vi "LINX - Blink (Advanced).vi"() -> ()   [LabVIEW 2020]
doc: "Automatically blink and LED attached to a digital output channel of a LINX device."
uses:
  vi.lib/MakerHub/LINX/Public/Peripherals/Digital/Digital Write 1 Chan.vi
  vi.lib/MakerHub/LINX/Public/Peripherals/Digital/Digital Write N Chans.vi
  vi.lib/MakerHub/LINX/Private/Local IO/LinxDigitalWrite.vi
  vi.lib/MakerHub/LINX/Public/Utilities/Check Channel.vi
  vi.lib/MakerHub/LINX/Public/Utilities/Open Serial.vi
  vi.lib/MakerHub/LINX/Private/Utilties/Generate Error.vi
  vi.lib/MakerHub/LINX/LMH-LINX.lvlib
  vi.lib/MakerHub/LINX/Private/Device/Device.lvlib
panel:
  out "LED Value":bool
  in  "Digital Output Channel":u8=13
  in  "Serial Port":refnum<visa-resource-name>
  out "Loop Rate (Hz)":u32
  in  "Stop Button":bool
  # "Circuit Schematic"
  # "LINX Device Settings"
  # "LED Value"
  # "Blink (Serial Interface)\n\nThis example demonstrates how to blink an LED on a LINX device connected to \nthe host computer using USB / Serial.\n\nInstructions\n1. Select the Serial Port associated with the LINX Device.\n2. Select the Digital Pin connected to the LED.\n3. Click the Run Arrow."
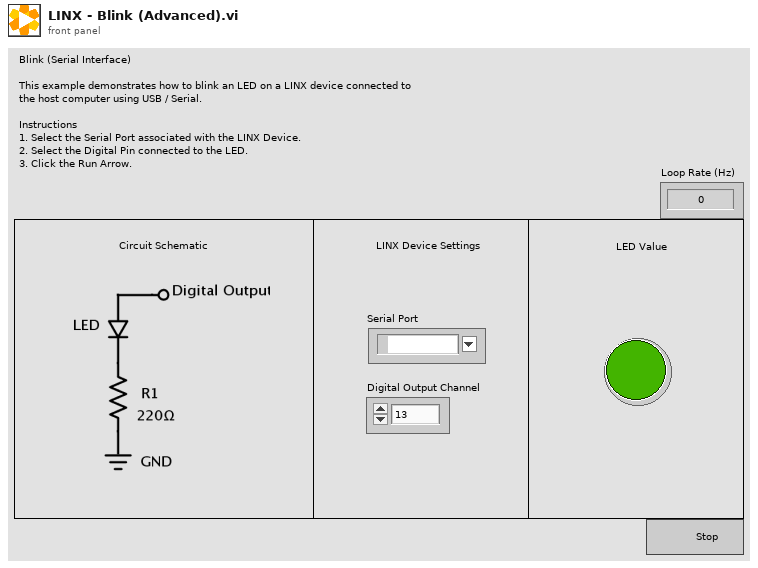
[diagram p1: front panel]
types:
  T1 = typedef "LMH-LINX.lvlib/LINX Ref.ctl" = cluster{"IO":T2, "Interface":T3, "LINX Device Config":T4}
  T2 = typedef "LMH-LINX.lvlib/Platform.ctl" = enum16{"Remote", "Local"}
  T3 = typedef "LMH-LINX.lvlib/Interface.ctl" = enum16{"Serial", "TCP"}
  T4 = typedef "Device.lvlib/LINX Device Config.ctl" = cluster{"Interface":T3, "COM Port":refnum<visa-resource-name>, "TCP Configuration":T5, "Device Family":u8, "Device ID":u8, "Device Name":string, "TCP Ref":refnum<k5>, "Channels":T6}
  T5 = typedef "Device.lvlib/TCP Config.ctl" = cluster{"IP Address":string, "Port":u16}
  T6 = typedef "LMH-LINX.lvlib/Channels.ctl" = cluster{"DI":u8[], "DO":u8[], "AI":u8[], "AO":u8[], "PWM":u8[], "QE":u8[], "UART":u8[], "I2C 2":u8[], "SPI":u8[], "CAN":u8[], "Servo":u8[], "AI Ref (V)":dbl, "AI Resolution (Bits)":u8, "AO Ref (V)":dbl, "AO Resolution (Bits)":u8}
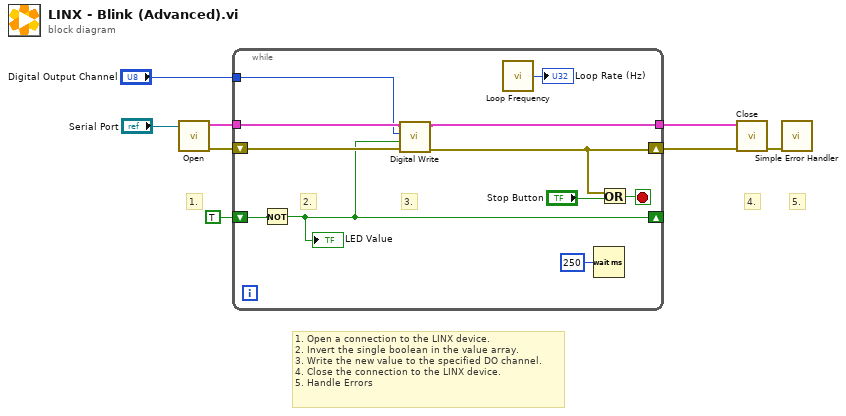
[diagram p0: block diagram]
diagram:
  # "1. Open a connection to the LINX device.\n2. Invert the single boolean in the value array.\n3. Write the new value to the specified DO channel.\n4. Close the connection to the LINX device.\n5. Handle Errors"
  # "5."
  # "4."
  # "1."
  n1 = call-poly "Open.vi"("Serial Port"="Serial Port") -> ("Error Out"=w7:errorcluster, "LINX Resource"=w8:T1)  [unwired: 8 in, 1 out]
  n2 = while {
    tunnel: w8 -> [w16]
    tunnel: [w15] -> w6
    shift-right: [w13] -> w5
    shift-left: w7 -> [w14]
    shift-right: [w9] -> _
    shift-left: TRUE -> [w10]
    tunnel: "Digital Output Channel" -> [w11]
    stop <- w19 stop-if-true
    # "2."
    # "3."
    n3 = Not(x=w10) -> (.not. x?=w9:bool)
    "LED Value" <- w9
    n4 = call-poly "Digital Write.vi"("Error In"=w14, "Output Value"=w9, "DO Channel"=w11, "LINX Resource"=w16) -> ("Error Out"=w13:errorcluster, "LINX Resource"=w15:T1)  [unwired: 6 in]
    n5 = call "Loop Frequency.vi"() -> ("Loop Rate (Hz)"=→"Loop Rate (Hz)":u32)
    n6 = Wait (ms)(milliseconds to wait=u32 250) -> ()  [unwired: 1 out]
    n7 = Or(x=w13, y="Stop Button") -> (x .or. y?=w19:bool)
  }
  n8 = call "Close.vi"("Error In"=w5, "LINX Resource"=w6) -> ("Error Out"=w3:errorcluster)  [unwired: 9 in]
  n9 = call <vilib>:"Simple Error Handler.vi"("error in (no error)"=w3) -> ()  [unwired: 4 in, 5 out]
